vi "Wait Timer mS.vi"(3 "Boolean In":bool, 4 "Timer":u32) -> (5 "Boolean Out":bool)   [LabVIEW 2014]
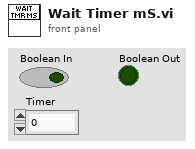
[diagram p1: front panel]
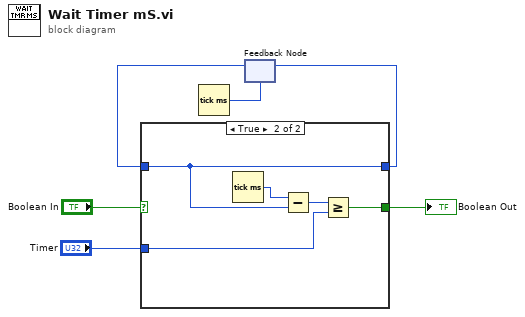
[diagram p0: block diagram]
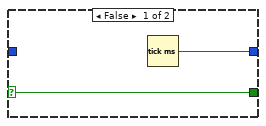
[diagram p2: hidden frame]
diagram:
  n1 = Tick Count (ms)() -> (millisecond timer value=w1:u32)
  n2 = feedback #1(w1) -> (w3:u32)
  n3 = case shown="True" "Boolean In" {
    selector: "Boolean In" -> [w8 _]
    tunnel: "Timer" -> [_ w9]
    tunnel: [w7 w10] -> w4
    tunnel: w3 -> [_ w10]
    tunnel: [w8 w11] -> w2
    frame False {
      n4 = Tick Count (ms)() -> (millisecond timer value=w7:u32)
    }
    frame True {
      n5 = Tick Count (ms)() -> (millisecond timer value=w13:u32)
      n6 = Subtract(x=w13, y=w10) -> (x-y=w12:u32)
      n7 = Greater Or Equal?(x=w12, y=w9) -> (x >= y?=w11:bool)
    }
  }
  "Boolean Out" <- w2
  n8 = feedback-in #1(w4) -> ()
